vi "Write PS Dataset Msg.vi"(10 "Power Supply.lvlib:PS Dataset Msg.lvclass":refnum<class "PS Dataset Msg.lvclass">, 11 "Power Supply in":refnum<class "Power Supply.lvclass">) -> (3 "Power Supply out":refnum<class "Power Supply.lvclass">)   [LabVIEW 2019, in "Power Supply.lvlib" / "Power Supply.lvclass"]
uses:
  Power Supply.lvclass
  Power Supply Messages/PS Dataset Msg/PS Dataset Msg.lvclass
  Power Supply.lvclass/Power Supply.ctl
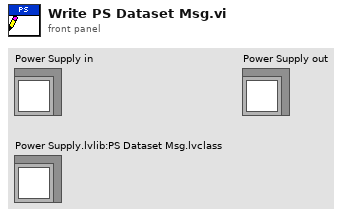
[diagram p1: front panel]
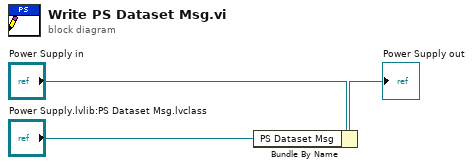
[diagram p0: block diagram]
diagram:
  n1 = Bundle By Name(cluster="Power Supply in", "PS Dataset Msg"="Power Supply.lvlib:PS Dataset Msg.lvclass") -> (→"Power Supply out":refnum<class "Power Supply.lvclass">)
